vi "TCP Read.vi"(7 "mode (standard)":T1(ring), 8 "error in (no error)":errorcluster, 9 "timeout ms (25000)":i32=25000, 10 "bytes to read":i32, 11 "TCP in":refnum<class "TCP.lvclass">) -> (0 "error out":errorcluster, 2 "data out":string, 3 "TCP out":refnum<class "TCP.lvclass">)   [LabVIEW 2013, in "TCP.lvclass"]
doc: "Reads a number of bytes from a TCP network connection"
uses:
  TCP.lvclass
  TCP.lvclass/TCP.ctl
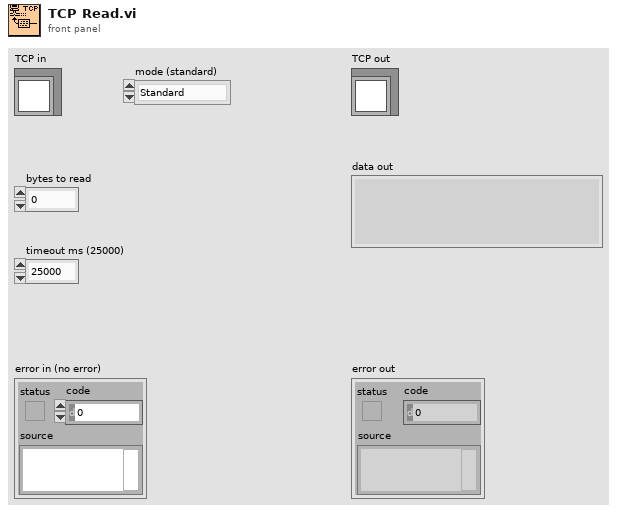
[diagram p1: front panel]
types:
  T1 = enum16{"Standard", "Buffered", "CRLF", "Immediate"}
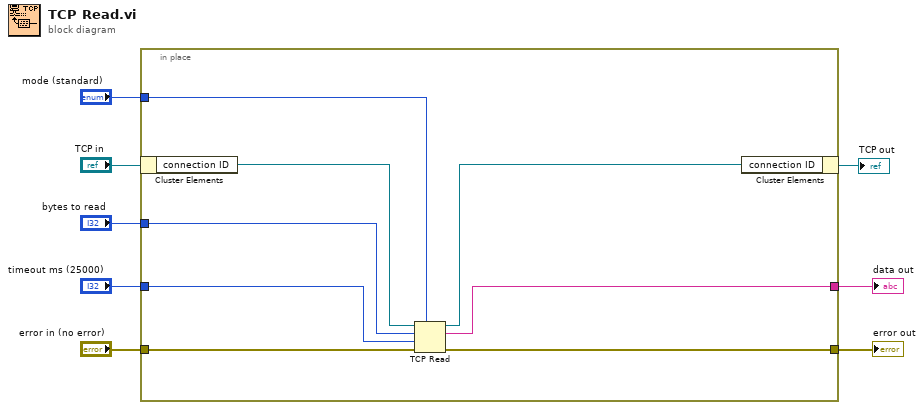
[diagram p0: block diagram]
diagram:
  n1 = in-place {
    in-place-border: "bytes to read" -> [w14]
    in-place-border: "timeout ms (25000)" -> [w13]
    in-place-border: "error in (no error)" -> [w12]
    in-place-border: "mode (standard)" -> [w11]
    in-place-border: [w10] -> w2
    in-place-border: [w9] -> w1
    n2 = in-place-cluster #1("TCP in") -> ("connection ID"=w16:refnum<k5>)
    n3 = TCP Read(connection ID=w16, bytes to read=w14, error in (no error)=w12, 7:w11, 9:w13) -> (connection ID out=w15:refnum<k5>, data out=w10:string, error out=w9:errorcluster)
    n4 = in-place-cluster #1("connection ID"=w15) -> (→"TCP out":refnum<class "TCP.lvclass">)
  }
  "error out" <- w1
  "data out" <- w2
